vi "Actor Core.vi"(8 "error in":errorcluster, 11 "TCP_Client in":refnum<class "TCP_Client.lvclass">) -> (0 "error out":errorcluster, 3 "Actor out":refnum<class "Actor.lvclass">)   [LabVIEW 2023, in "TCP_Client.lvlib" / "TCP_Client.lvclass"]
doc: "(<B>Filename</B>: Actor Framework.lvlib:Actor.lvclass:Actor Core.vi)\n\nReceives messages to the actor, reacts to them, and initiates any error handling that may shut the actor down.\n\nDescendant classes may override this VI to append parallel tasks for the actor to complete while it handles messages. Overrides use the Call Parent Class Method node."
uses:
  TCP_Client.lvclass
  C:/Program Files (x86)/National Instruments/LabVIEW 2023/vi.lib/ActorFramework/Actor/Actor.lvclass
  <vilib>/ActorFramework/Actor/Actor.lvclass
  TypeDefinitions/ActorCoreFPcontrols.ctl
  TCP_Client.lvclass/TCP_Client.ctl
  <vilib>/ActorFramework/Actor/Actor.lvclass/Actor.ctl
  <vilib>/ActorFramework/Message Enqueuer/Message Enqueuer.lvclass/Message Enqueuer.ctl
  TCP_Client Messages/SendMessageToServer Msg/SendMessageToServer Msg.lvclass/SendMessageToServer Msg.ctl
  TCP_Client Messages/Upload Msg/Upload Msg.lvclass/Upload Msg.ctl
  <vilib>/ActorFramework/Message Enqueuer/Init from Existing Queue.vi
  <vilib>/ActorFramework/Message Enqueuer/Enqueue.vi
  <vilib>/ActorFramework/Stop Msg/Stop Msg.lvclass
  C:/Program Files (x86)/National Instruments/LabVIEW 2023/vi.lib/ActorFramework/Message/Message.lvclass
  TCP_Client Messages/SendMessageToServer Msg/SendMessageToServer Msg.lvclass
  TCP_Client Messages/Upload Msg/Upload Msg.lvclass
  TCP_Client Messages/Connect Msg/Connect Msg.lvclass
  <vilib>/ActorFramework/Message Priority Queue/Priority Enqueue.vi
  <vilib>/ActorFramework/Message Enqueuer/Message Enqueuer.lvclass
panel:
  in  "Upload Button":bool
  in  "File to upload":path
  out "Error log filenumber":u32
  out "Error log file":path
  out "Error Count":u32
  in  "Local Port":u16
  in  "Remote Port":u16=30000
  in  "Connect Button":bool
  in  "Server address":string="127.0.0.1"
  in  "Shut down server  Button":bool
  in  "Close Button":bool
  in  "Send Button":bool
  in  "Messages to server":string
  out "Messages from server":string
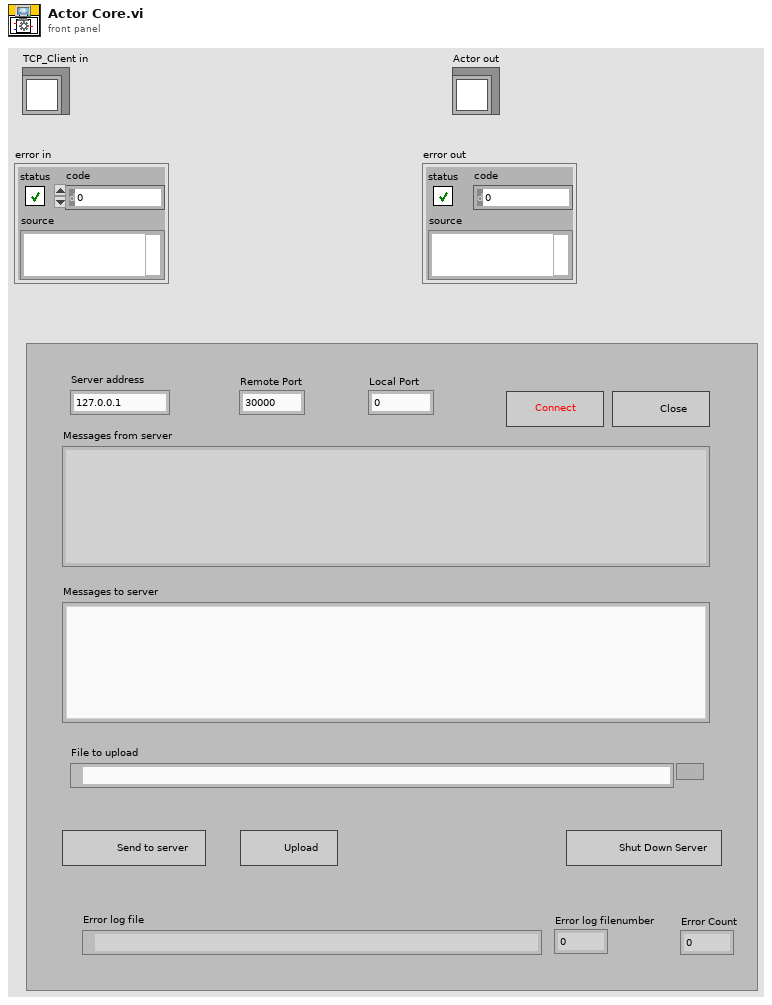
[diagram p1: front panel]
types:
  T1 = enum8{"Enabled", "Disabled", "Disabled and Grayed Out"}
  T2 = typedef "TCP_Client.lvlib/TCP_Client.lvclass/ActorCoreFPcontrols.ctl" = cluster{"Messages from server":refnum<vi>, "Messages to server":refnum<vi>, "Server address":refnum<vi>, "Remote Port":refnum<vi>, "Local Port":refnum<vi>, "Connect Button":refnum<vi>, "Send Button":refnum<vi>, "Error Count":refnum<vi>, "Error log filenumber":refnum<vi>, "Error log file":refnum<vi>, "Shut down server  Button":refnum<vi>, "Upload Button":refnum<vi>, "File to upload":refnum<vi>}
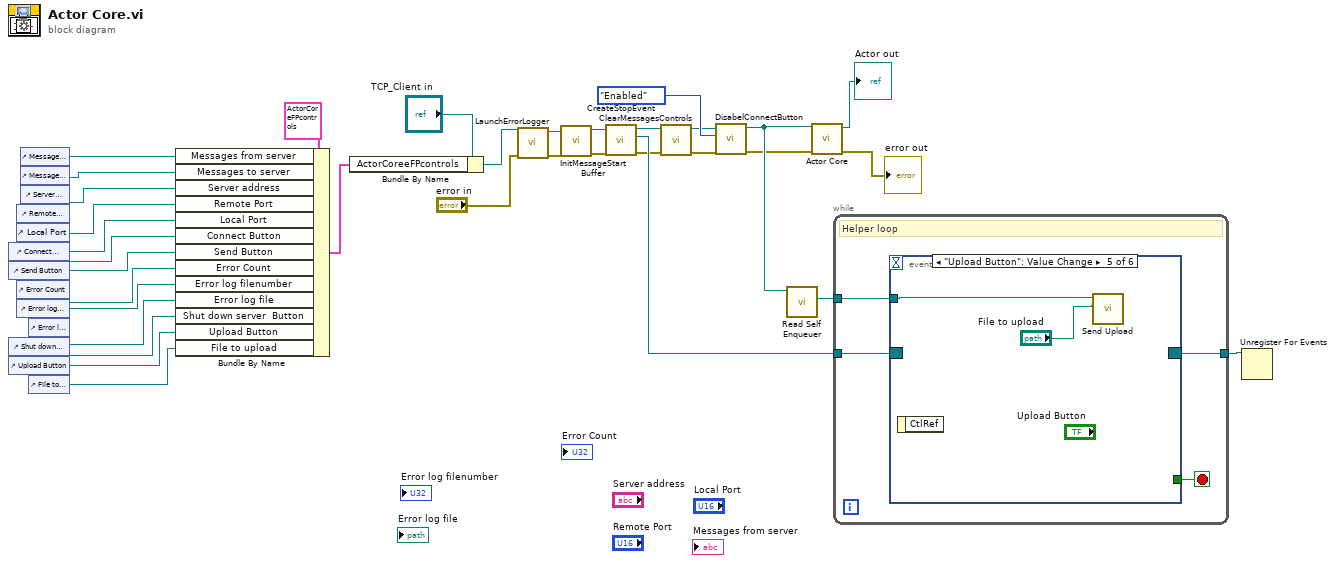
[diagram p0: block diagram]
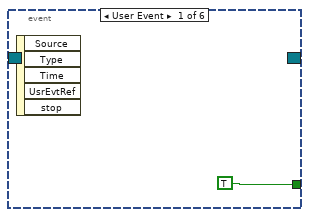
[diagram p2: hidden frame]
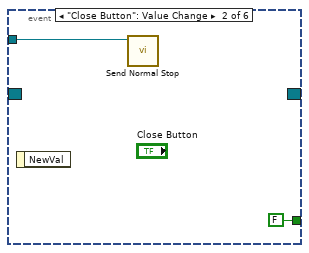
[diagram p3: hidden frame]
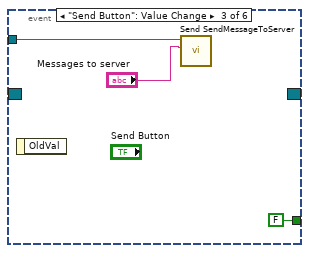
[diagram p4: hidden frame]
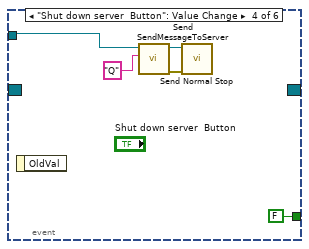
[diagram p5: hidden frame]
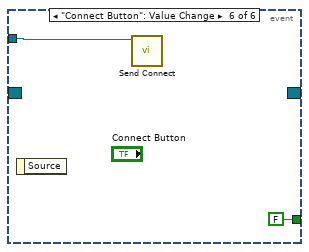
[diagram p6: hidden frame]
diagram:
  n1 = control-ref of="Connect Button"() -> (w21:refnum<vi>)
  n2 = control-ref of="Send Button"() -> (w20:refnum<vi>)
  n3 = control-ref of="Shut down server  Button"() -> (w3:refnum<vi>)
  n4 = control-ref of="Upload Button"() -> (w2:refnum<vi>)
  n5 = control-ref of="Remote Port"() -> (w25:refnum<vi>)
  n6 = control-ref of="Local Port"() -> (w24:refnum<vi>)
  n7 = control-ref of="Error Count"() -> (w6:refnum<vi>)
  n8 = control-ref of="Error log filenumber"() -> (w5:refnum<vi>)
  n9 = control-ref of="Messages from server"() -> (w29:refnum<vi>)
  n10 = control-ref of="Messages to server"() -> (w28:refnum<vi>)
  n11 = control-ref of="Server address"() -> (w26:refnum<vi>)
  n12 = control-ref of="Error log file"() -> (w4:refnum<vi>)
  n13 = control-ref of="File to upload"() -> (w1:refnum<vi>)
  n14 = Bundle By Name(cluster=T2 {"Messages from server"=refnum, "Messages to server"=refnum, "Server address"=refnum, "Remote Port"=refnum, "Local Port"=refnum, "Connect Button"=refnum, "Send Button"=refnum, "Error Count"=refnum, "Error log filenumber"=refnum, "Error log file"=refnum, "Shut down server  Button"=refnum, "Upload Button"=refnum, "File to upload"=refnum} ("Cluster"), "Messages from server"=w29, "Messages to server"=w28, "Server address"=w26, "Remote Port"=w25, "Local Port"=w24, "Connect Button"=w21, "Send Button"=w20, "Error Count"=w6, "Error log filenumber"=w5, "Error log file"=w4, "Shut down server  Button"=w3, "Upload Button"=w2, "File to upload"=w1) -> (w27:T2)
  n15 = Bundle By Name(cluster="TCP_Client in", "ActorCoreeFPcontrols"=w27) -> (w12:refnum<class "TCP_Client.lvclass">)
  n16 = call "LaunchErrorLogger.vi"("error in (no error)"="error in", "TCP_Client in"=w12) -> ("error out"=w10:errorcluster, "TCP_Client out"=w13:refnum<class "TCP_Client.lvclass">)  [unwired: 8 in]
  n17 = call "InitMessageStartBuffer.vi"("error in (no error)"=w10, "TCP_Client in"=w13) -> ("error out"=w9:errorcluster, "TCP_Client out"=w23:refnum<class "TCP_Client.lvclass">)  [unwired: 8 in]
  n18 = call "CreateStopEvent.vi"("error in (no error)"=w9, "TCP_Client in"=w23) -> ("error out"=w14:errorcluster, "Event Registration Refnum"=w33:refnum<event-registration>, "TCP_Client out"=w15:refnum<class "TCP_Client.lvclass">)  [unwired: 7 in]
  n19 = call "ClearMessagesControls.vi"("error in (no error)"=w14, "TCP_Client in"=w15) -> ("error out"=w16:errorcluster, "TCP_Client out"=w17:refnum<class "TCP_Client.lvclass">)  [unwired: 8 in]
  n20 = call "DisabelConnectButton.vi"("error in (no error)"=w16, "Connect button Disabled"=T1."Enabled", "TCP_Client in"=w17) -> ("error out"=w8:errorcluster, "TCP_Client out"=w19:refnum<class "TCP_Client.lvclass">)  [unwired: 7 in]
  n21 = call <vilib>:"Read Self Enqueuer.vi"("Actor"=w19) -> ("Self Enqueuer"=w31:refnum<class "Message Enqueuer.lvclass">)  [unwired: 10 in]
  n22 = call-parent "Actor Core.vi"("error in"=w8, "Actor in"=w19) -> ("error out"=→"error out":errorcluster, "Actor out"=→"Actor out":refnum<class "Actor.lvclass">)  [unwired: 8 in]
  n23 = while {
    tunnel: w33 -> [w38]
    tunnel: [w37] -> w32
    tunnel: w31 -> [w35]
    stop <- w36 stop-if-true
    # "Helper loop"
    n24 = event shown="[4] \"Upload Button\": Value Change" {
      selector: w38 -> [_ _ _ _ _ _]
      dyn-events: [_ _ _ _ _ _] -> w37
      timeout: _ -> [_ _ _ _ _ _]
      tunnel: [TRUE FALSE FALSE FALSE _ FALSE] -> w36
      tunnel: w35 -> [_ w41 w43 w48 w51 w52]
      event User Event {
        n25 = event-data() -> ()  [unwired: 1 in, 5 out]
      }
      event "Close Button": Value Change {
        n26 = event-data() -> ()  [unwired: 1 in, 1 out]
        n27 = call <vilib>:"Send Normal Stop.vi"("Message Enqueuer"=w41) -> ()  [unwired: 10 in, 1 out]
      }
      event "Send Button": Value Change {
        n28 = event-data() -> ()  [unwired: 1 in, 1 out]
        n29 = call "Send SendMessageToServer.vi"("Message"="Messages to server", "Message Enqueuer"=w43) -> ()  [unwired: 8 in, 2 out]
      }
      event "Shut down server  Button": Value Change {
        n30 = event-data() -> ()  [unwired: 1 in, 1 out]
        n31 = call "Send SendMessageToServer.vi"("Message"="Q", "Message Enqueuer"=w48) -> ("error out"=w46:errorcluster, "Message Enqueuer out"=w45:refnum<class "Message Enqueuer.lvclass">)  [unwired: 8 in]
        n32 = call <vilib>:"Send Normal Stop.vi"("error in (no error)"=w46, "Message Enqueuer"=w45) -> ()  [unwired: 9 in, 1 out]
      }
      event "Upload Button": Value Change {
        n33 = event-data() -> ()  [unwired: 1 in, 1 out]
        n34 = call "Send Upload.vi"("File"="File to upload", "Message Enqueuer"=w51) -> ()  [unwired: 8 in, 2 out]
      }
      event "Connect Button": Value Change {
        n35 = event-data() -> ()  [unwired: 1 in, 1 out]
        n36 = call "Send Connect.vi"("Message Enqueuer"=w52) -> ()  [unwired: 9 in, 2 out]
      }
    }
  }
  n37 = Unregister For Events(event registration refnum=w32) -> ()  [unwired: 1 in, 1 out]
